vi "TP_ShouldFlipAcceleration.vi"(9 "Constraints":T1, 10 "Goal":T2, 11 "Initial":T2) -> (3 "Is Accel Flipped?":bool)   [LabVIEW 2018, in "TrapezoidalProfile.lvclass"]
uses:
  TrapezoidalProfile.lvclass
  State.ctl
  Constraints.ctl
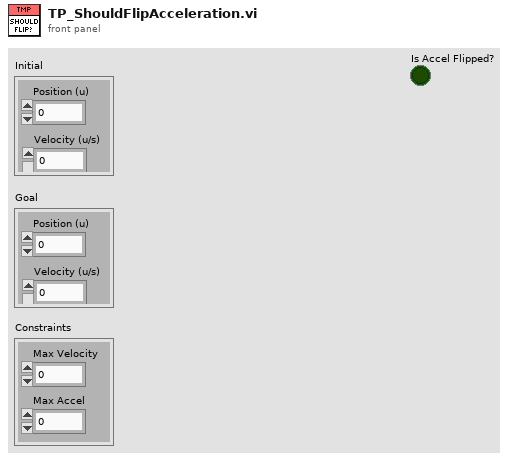
[diagram p1: front panel]
types:
  T1 = typedef "TrapezoidalProfile.lvclass/Constraints.ctl" = cluster{"Max Velocity":dbl, "Max Accel":dbl}
  T2 = typedef "TrapezoidalProfile.lvclass/State.ctl" = cluster{"Position (u)":dbl, "Velocity (u/s)":dbl}
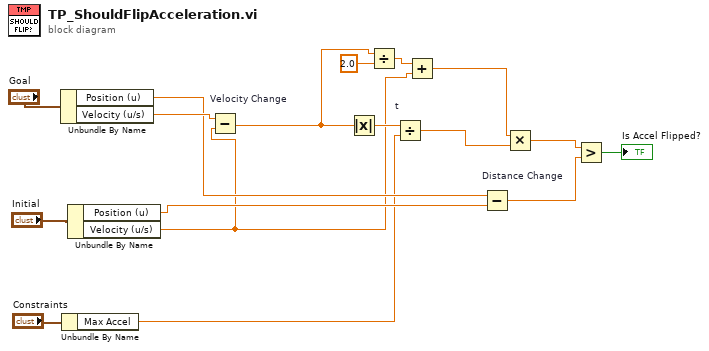
[diagram p0: block diagram]
diagram:
  n1 = Unbundle By Name("Goal") -> ("Position (u)"=w14:dbl, "Velocity (u/s)"=w15:dbl)
  n2 = Unbundle By Name("Constraints") -> ("Max Accel"=w10:dbl)
  n3 = Unbundle By Name("Initial") -> ("Position (u)"=w13:dbl, "Velocity (u/s)"=w6:dbl)
  n4 = Subtract "Velocity Change"(x=w15, y=w6) -> (x-y=w8:dbl)
  n5 = Absolute Value(x=w8) -> (abs(x)=w11:dbl)
  n6 = Divide(x=w8, y=2.0) -> (x/y=w7:dbl)
  n7 = Divide "t"(x=w11, y=w10) -> (x/y=w5:dbl)
  n8 = Add(x=w7, y=w6) -> (x+y=w4:dbl)
  n9 = Subtract "Distance Change"(x=w14, y=w13) -> (x-y=w2:dbl)
  n10 = Multiply(x=w4, y=w5) -> (x*y=w3:dbl)
  n11 = Greater?(x=w3, y=w2) -> (0:→"Is Accel Flipped?":bool)
